vi "WrittingSpectrumAndImageAttributes.vi"() -> ()   [LabVIEW 2013, in "examples.lvlib"]
uses:
  examples.lvlib
  vis/lv-2013/tango_vi.llb/ReadULongImageAttribute.vi
  vis/lv-2013/tango_vi.llb/WriteULongImageAttribute.vi
  vis/lv-2013/tango_vi.llb/ReadDoubleImageAttribute.vi
  vis/lv-2013/tango_vi.llb/WriteDoubleImageAttribute.vi
  vis/lv-2013/tango_vi.llb/ReadFloatImageAttribute.vi
  vis/lv-2013/tango_vi.llb/WriteFloatImageAttribute.vi
  vis/lv-2013/tango_vi.llb/ReadBooleanImageAttribute.vi
  vis/lv-2013/tango_vi.llb/WriteBooleanImageAttribute.vi
  vis/lv-2013/tango_vi.llb/ReadUCharImageAttribute.vi
  vis/lv-2013/tango_vi.llb/WriteUCharImageAttribute.vi
  vis/lv-2013/tango_vi.llb/ReadUShortImageAttribute.vi
  vis/lv-2013/tango_vi.llb/WriteUShortImageAttribute.vi
  vis/lv-2013/tango_vi.llb/WriteLongSpectrumAttribute.vi
  vis/lv-2013/tango_vi.llb/ReadLongSpectrumAttribute.vi
  vis/lv-2013/tango_vi.llb/ReadLongImageAttribute.vi
  vis/lv-2013/tango_vi.llb/WriteLongImageAttribute.vi
  vis/lv-2013/tango_vi.llb/WriteDoubleSpectrumAttribute.vi
  vis/lv-2013/tango_vi.llb/ReadDoubleSpectrumAttribute.vi
  vis/lv-2013/tango_vi.llb/WriteFloatSpectrumAttribute.vi
  vis/lv-2013/tango_vi.llb/ReadFloatSpectrumAttribute.vi
  vis/lv-2013/tango_vi.llb/ReadShortImageAttribute.vi
  vis/lv-2013/tango_vi.llb/WriteShortImageAttribute.vi
  vis/lv-2013/tango_vi.llb/WriteUCharSpectrumAttribute.vi
  vis/lv-2013/tango_vi.llb/ReadUCharSpectrumAttribute.vi
  vis/lv-2013/tango_vi.llb/WriteBooleanSpectrumAttribute.vi
  vis/lv-2013/tango_vi.llb/ReadBooleanSpectrumAttribute.vi
  vis/lv-2013/tango_vi.llb/WriteUShortSpectrumAttribute.vi
  vis/lv-2013/tango_vi.llb/ReadUShortSpectrumAttribute.vi
  vis/lv-2013/tango_vi.llb/WriteShortSpectrumAttribute.vi
  vis/lv-2013/tango_vi.llb/ReadShortSpectrumAttribute.vi
  vis/lv-2013/tango_vi.llb/tango.lvlib
panel:
  in  "TangoTest dev. name 3":string="tango/tangotest/1"
  out "Success-R":bool
  out "Success-Cmp 3":bool
  out "ULong Image R":u32[][](graph)
  out "Success-W":bool
  out "ULong Image W":u32[][](graph)
  out "Success-R":bool
  out "Success-Cmp":bool
  out "Double  Image R":dbl[][](graph)
  out "Success-W":bool
  out "Double Image W":dbl[][](graph)
  out "Success-R":bool
  out "Success-Cmp":bool
  out "Float Image R":sgl[][](graph)
  out "Success-W":bool
  out "Float Image W":sgl[][](graph)
  out "Success-R":bool
  out "Success-Cmp":bool
  out "Boolean  Image R":i16[][](graph)
  out "Success-W":bool
  out "Boolean Image W":i16[][](graph)
  out "Success-R":bool
  out "Success-Cmp":bool
  out "UChar Image R":u8[][](graph)
  out "Success-W":bool
  out "UChar Image W":u8[][](graph)
  out "Success-R":bool
  out "Success-Cmp":bool
  out "UShort Image R":u16[][](graph)
  out "Success-W":bool
  out "UShort Image W":u16[][](graph)
  out "Long Spectrum R":i32[](graph)
  out "Success-R":bool
  out "Success-Cmp":bool
  out "Success-W":bool
  out "Long  Spectrum W":i32[](graph)
  out "Success-R":bool
  out "Success-Cmp":bool
  out "Long Image R":i32[][](graph)
  out "Success-W":bool
  out "Long Image W":i32[][](graph)
  out "Double Spectrum R":dbl[](graph)
  out "Success-R":bool
  out "Success-Cmp":bool
  out "Success-W":bool
  out "Double  Spectrum W":dbl[](graph)
  out "Float Spectrum R":sgl[](graph)
  out "Success-R":bool
  out "Success-Cmp":bool
  out "Success-W":bool
  out "Float Spectrum W":sgl[](graph)
  out "Short Image R":i16[][](graph)
  out "Short Image W":i16[][](graph)
  out "Success-R":bool
  out "Success-Cmp 2":bool
  out "Success-W":bool
  out "error stack":string[](array[string])
  in  "TangoTest Device Name 5":string="tango/tangotest/1"
  in  "TangoTest Device Name 4":string="tango/tangotest/1"
  in  "TangoTest Device Name 3":string="tango/tangotest/1"
  in  "TangoTest Device Name 2":string="tango/tangotest/1"
  in  "TangoTest dev. name":string="sys/tg_test/1"
  out "UChar Spectrum R":u8[](graph)
  out "Success-R":bool
  out "Success-Cmp":bool
  out "Success-W":bool
  out "UChar Spectrum W":u8[](graph)
  out "Boolean Spectrum R":i16[](graph)
  out "Success-R":bool
  out "Success-Cmp":bool
  out "Success-W":bool
  out "Boolean Spectrum W":i16[](graph)
  out "UShort Spectrum R":u16[](graph)
  out "Success-R":bool
  out "Success-Cmp":bool
  out "Success-W":bool
  out "UShort Spectrum W":u16[](graph)
  out "Success-Cmp":bool
  out "Success-W":bool
  out "Short Spectrum R":i16[](graph)
  out "Success-R":bool
  out "Short Spectrum W":i16[](graph)
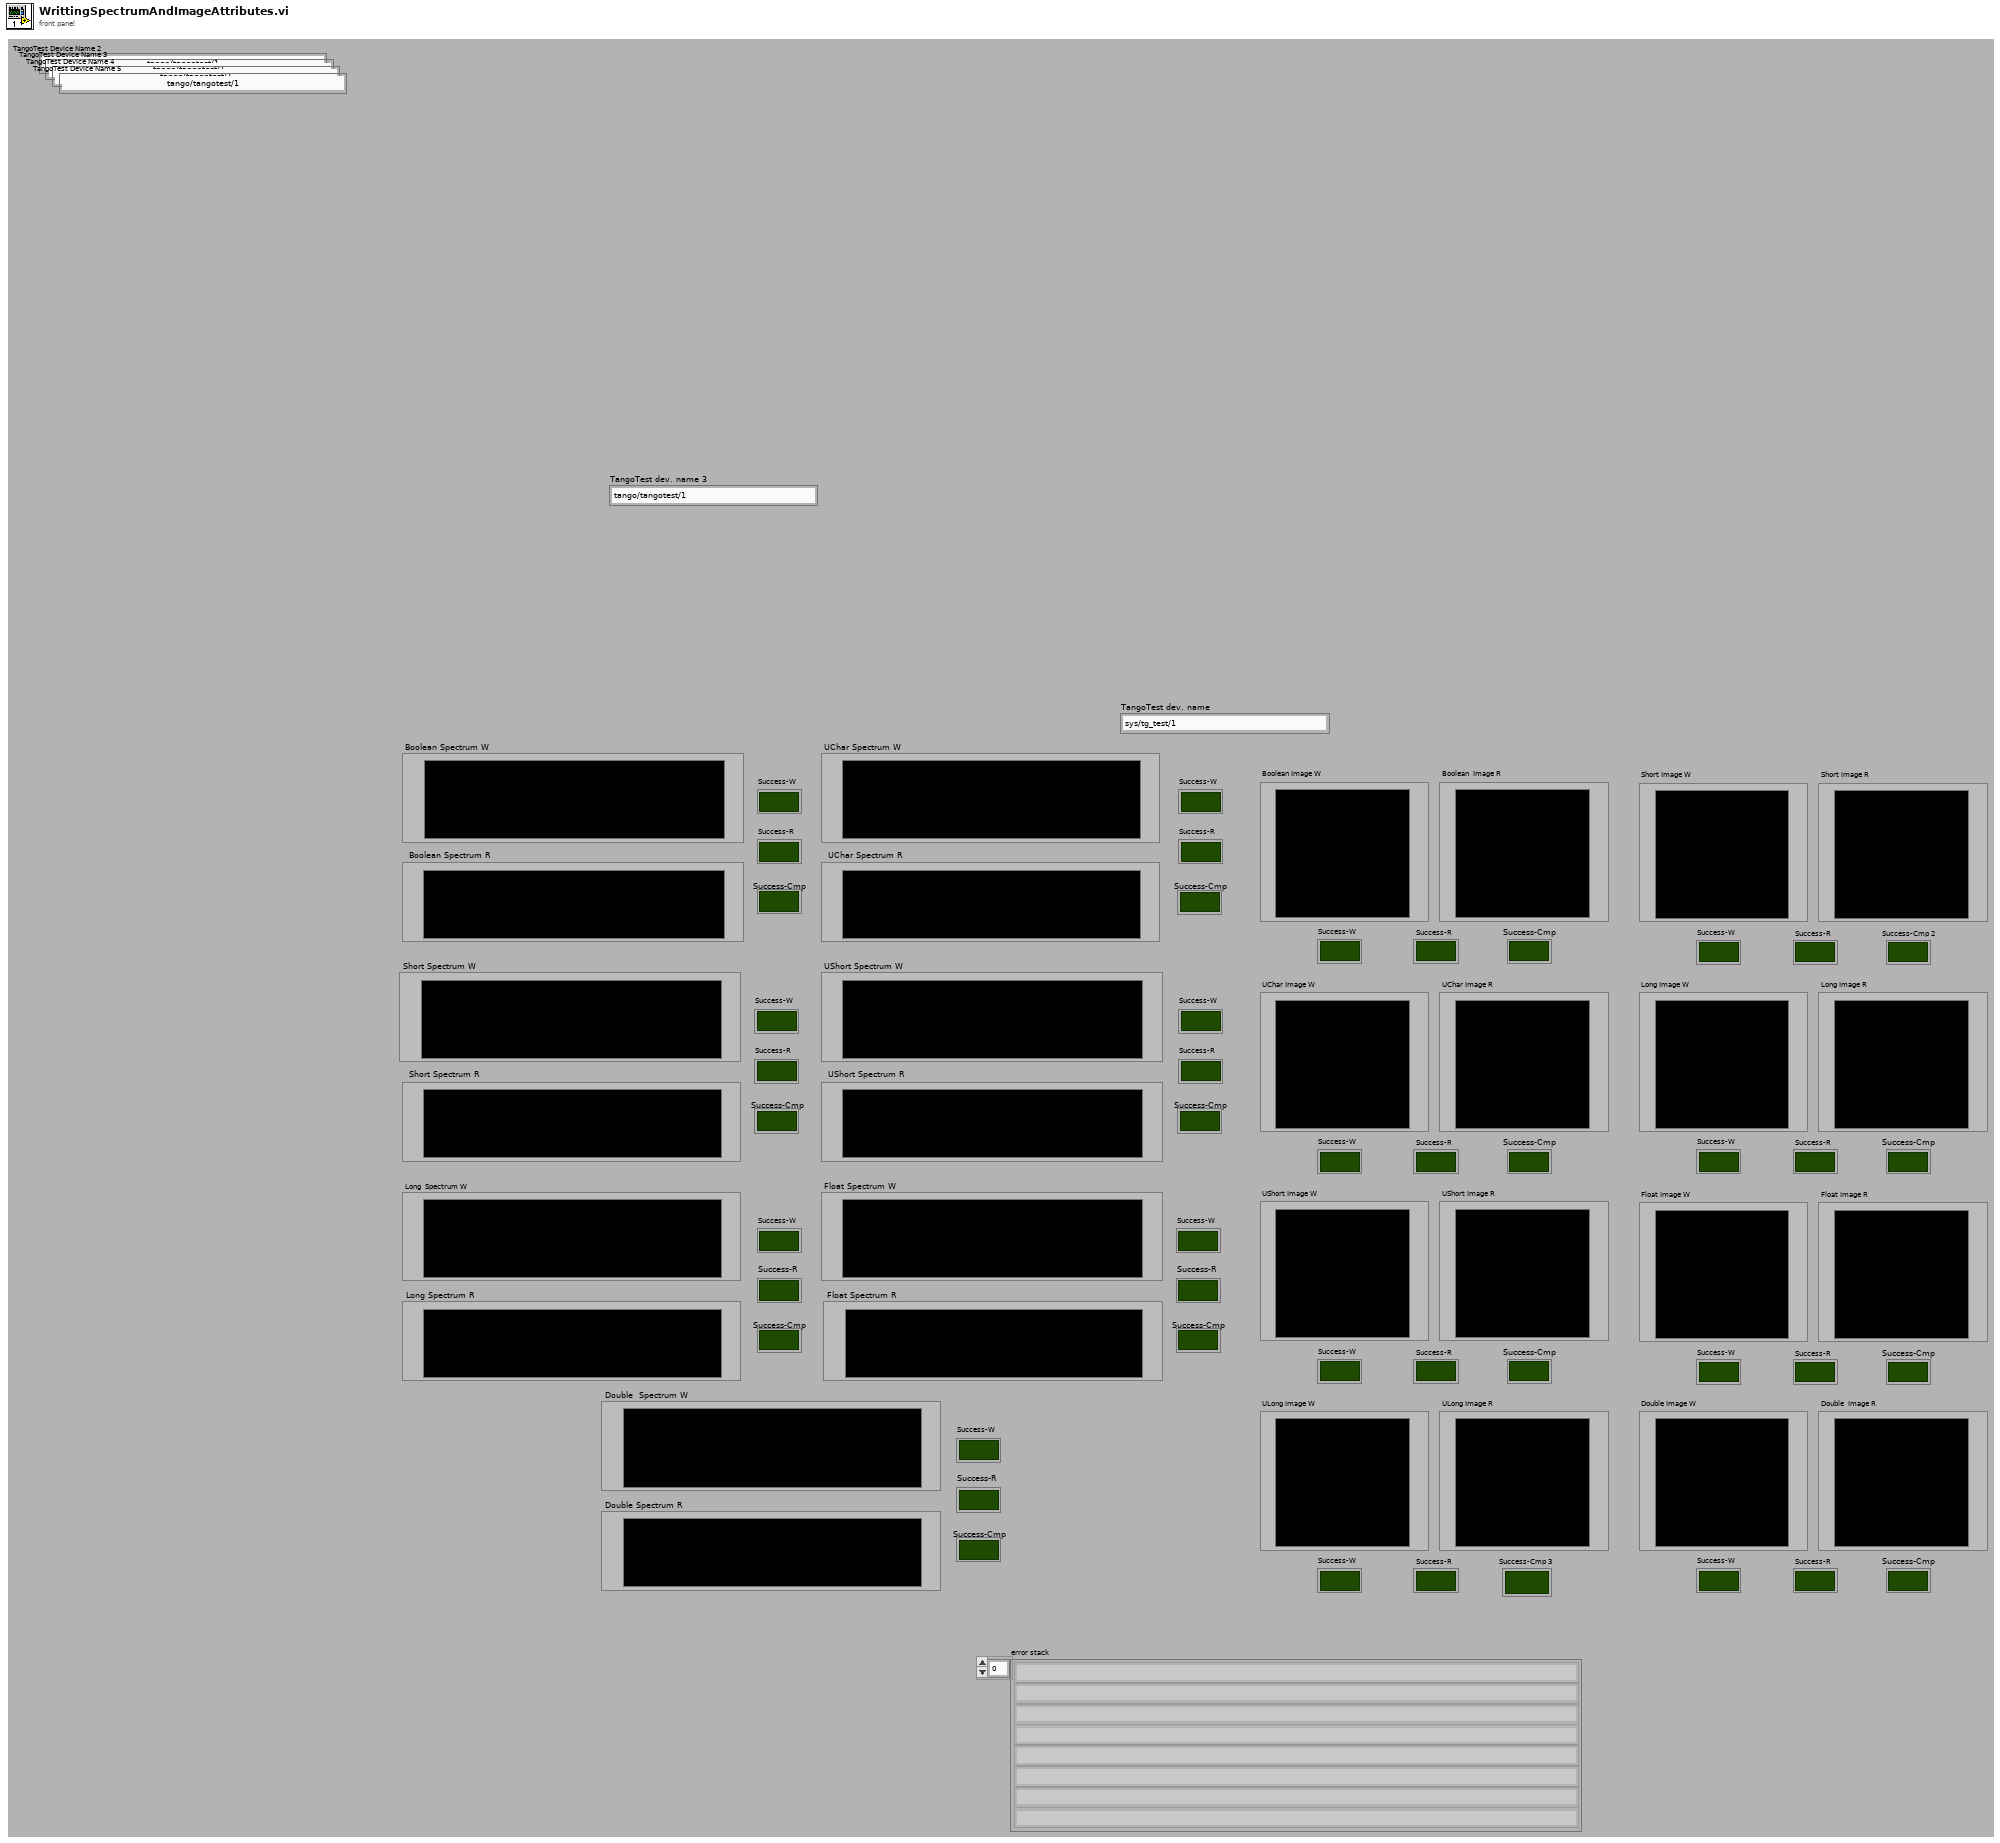
[diagram p1: front panel]
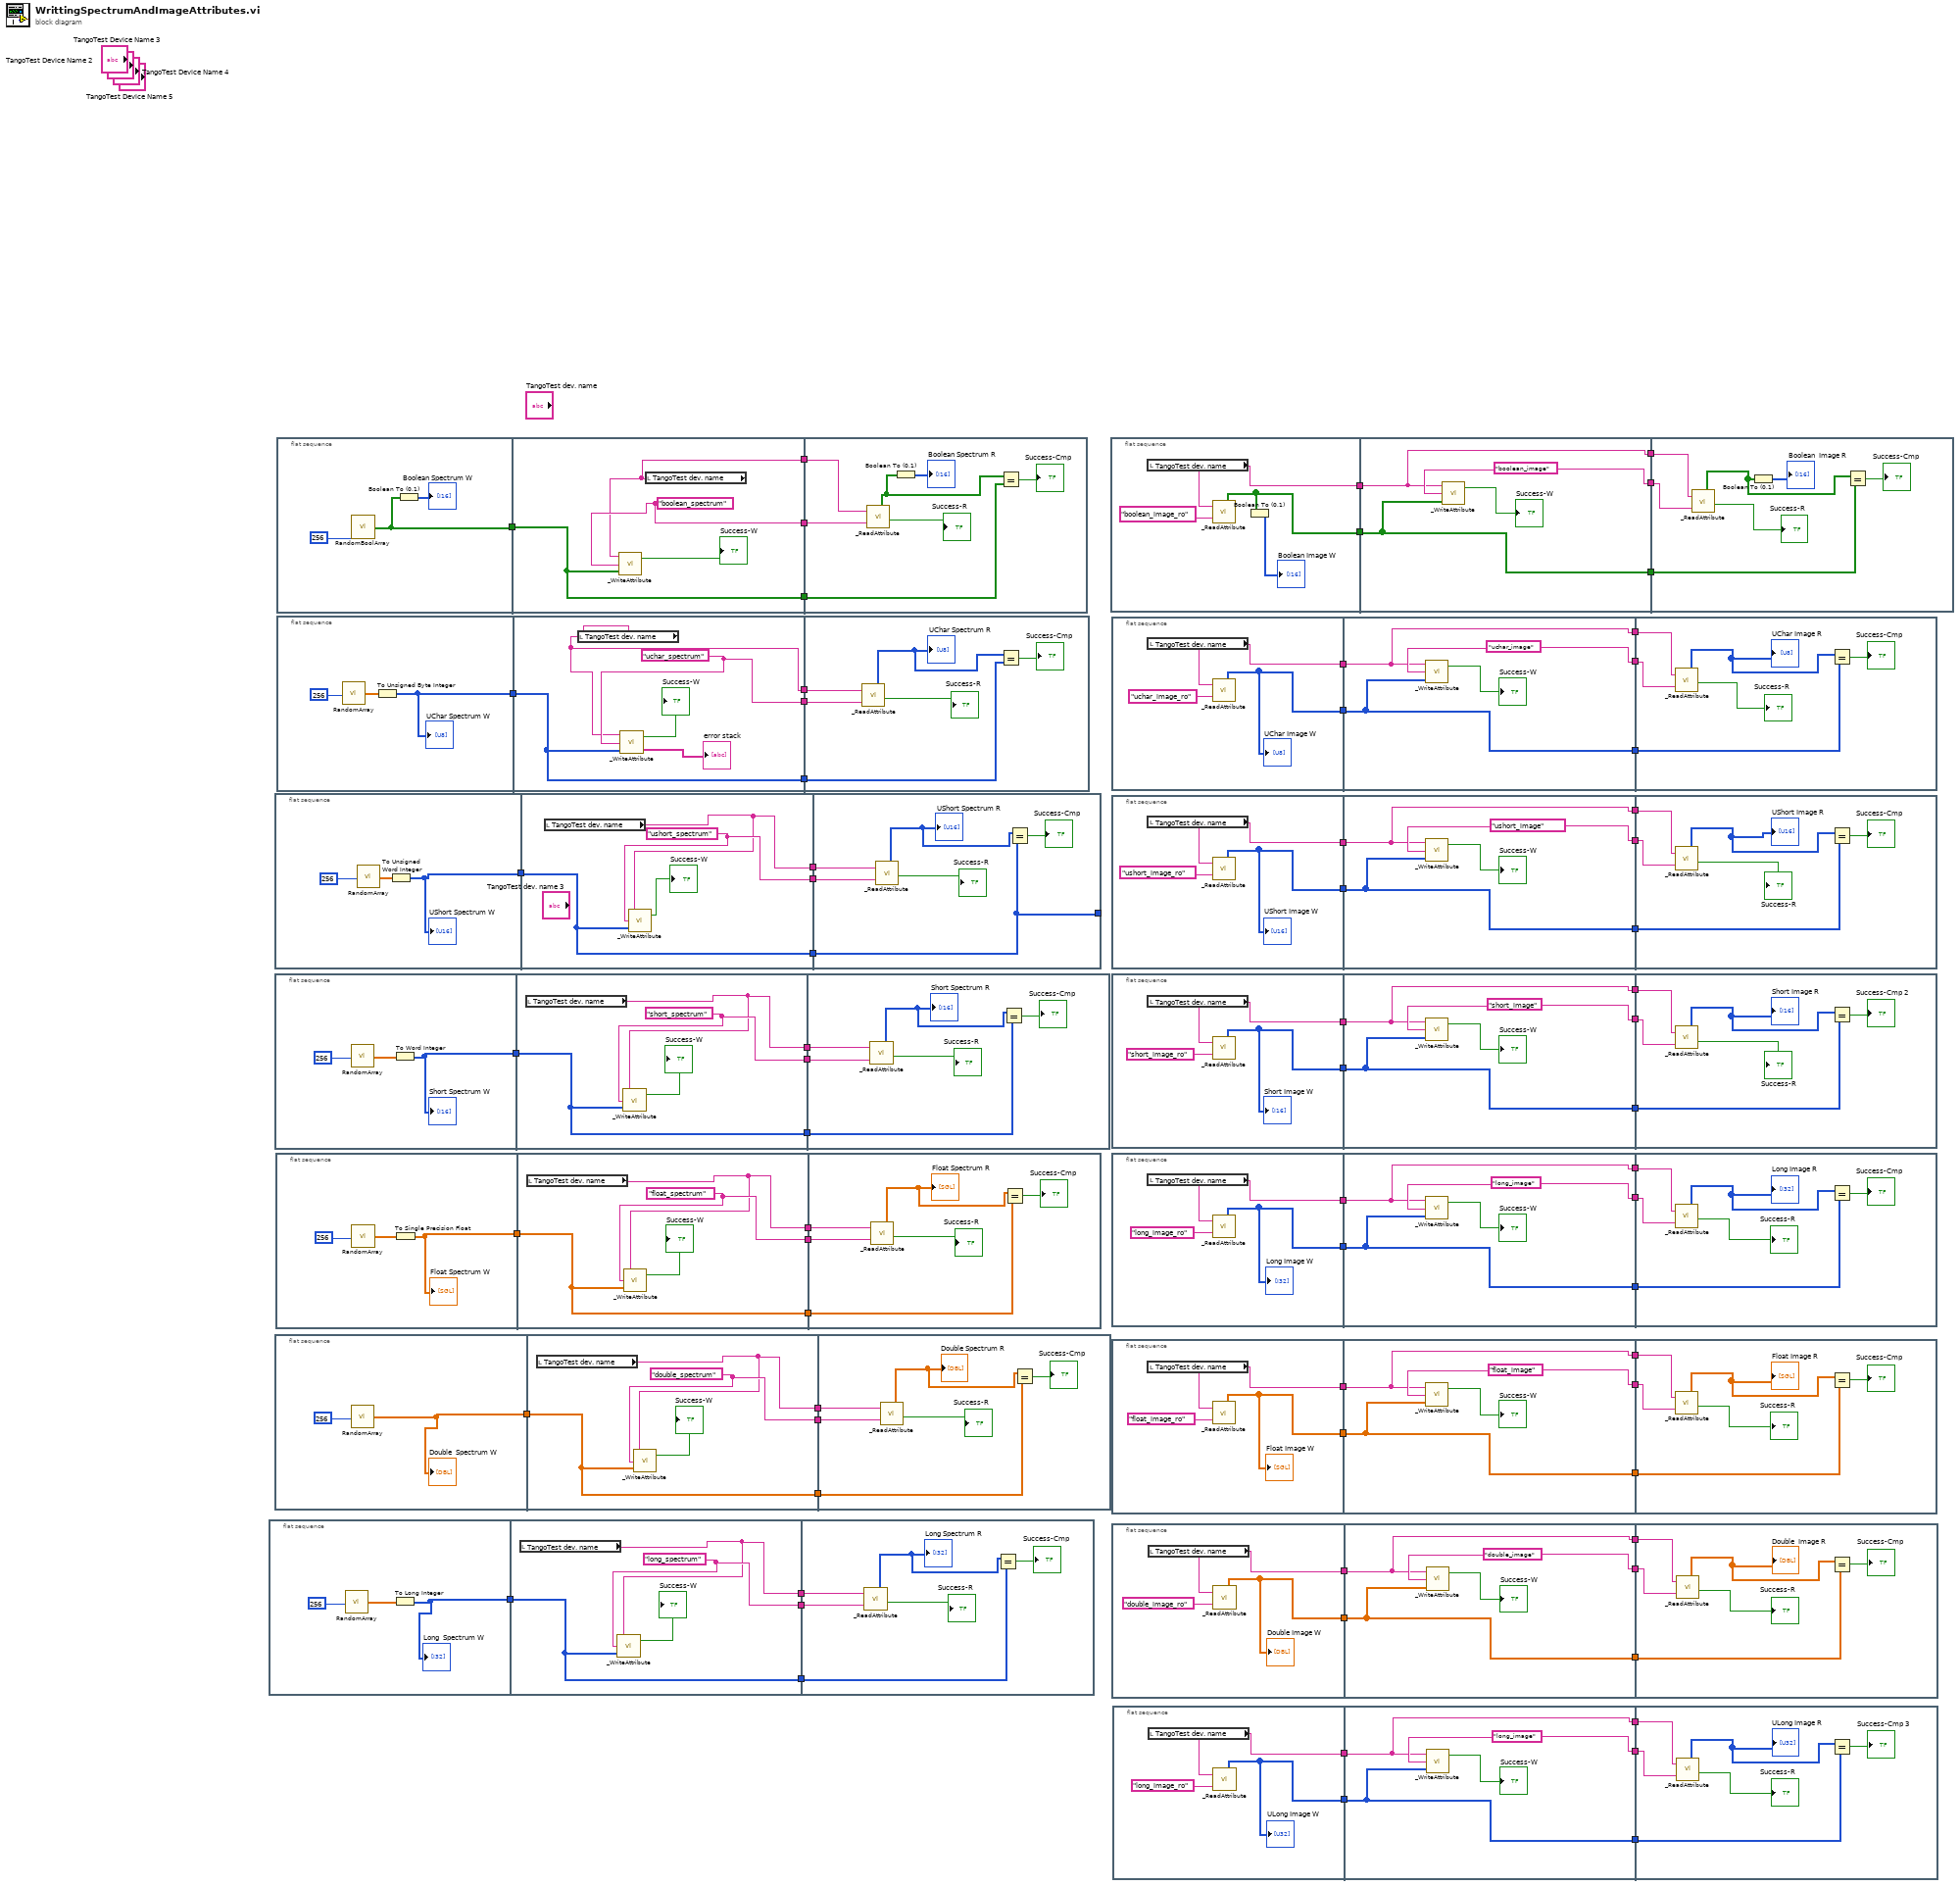
[diagram p0: block diagram]
diagram:
  n1 = flat-sequence {
    tunnel: [w69] -> w34
    tunnel: [w72] -> w33
    tunnel: [w74] -> w32
    tunnel: [w73] -> w31
    tunnel: w34 -> [w73]
    tunnel: w33 -> [w80]
    tunnel: w32 -> [w79]
    tunnel: w31 -> [w77]
    frame #0 {
      n2 = call "RandomArray.vi"("random array size"=256) -> ("random array"=w70:dbl[])  [unwired: 1 in]
      n3 = To Long Integer(number=w70) -> (32bit integer=w69:i32[])
      "Long  Spectrum W" <- w69
    }
    frame #1 {
      w74 = "long_spectrum" ("attribute name")
      n4 = local read "TangoTest dev. name"() -> (w72:string)
      n5 = call-poly "_WriteAttribute.vi"("value"=w73, "attribute name"=w74, "device name"=w72) -> ("success"=→"Success-W":bool)  [unwired: 1 out]
    }
    frame #2 {
      n6 = call-poly "_ReadAttribute.vi"("device name"=w80, "attribute name"=w79) -> ("value"=w78:i32[], "success"=→"Success-R":bool)  [unwired: 4 out]
      "Long Spectrum R" <- w78
      n7 = Equal?(x=w78, y=w77) -> (x = y?=→"Success-Cmp":bool)
    }
  }
  n8 = flat-sequence {
    tunnel: [w82] -> w64
    tunnel: [w86] -> w63
    tunnel: [w88] -> w62
    tunnel: [w87] -> w61
    tunnel: w64 -> [w87]
    tunnel: w63 -> [w93]
    tunnel: w62 -> [w92]
    tunnel: w61 -> [w89]
    tunnel: [w89] -> _
    frame #0 {
      n9 = call "RandomArray.vi"("random array size"=256) -> ("random array"=w83:dbl[])  [unwired: 1 in]
      n10 = To Unsigned Word Integer(number=w83) -> (unsigned 16bit integer=w82:u16[])
      "UShort Spectrum W" <- w82
    }
    frame #1 {
      w88 = "ushort_spectrum" ("attribute name")
      n11 = local read "TangoTest dev. name"() -> (w86:string)
      n12 = call-poly "_WriteAttribute.vi"("value"=w87, "attribute name"=w88, "device name"=w86) -> ("success"=→"Success-W":bool)  [unwired: 1 out]
    }
    frame #2 {
      n13 = call-poly "_ReadAttribute.vi"("device name"=w93, "attribute name"=w92) -> ("value"=w91:u16[], "success"=→"Success-R":bool)  [unwired: 4 out]
      "UShort Spectrum R" <- w91
      n14 = Equal?(x=w91, y=w89) -> (x = y?=→"Success-Cmp":bool)
    }
  }
  n15 = flat-sequence {
    tunnel: [w95] -> w65
    tunnel: [w98] -> w68
    tunnel: [w100] -> w67
    tunnel: [w99] -> w66
    tunnel: w65 -> [w99]
    tunnel: w68 -> [w106]
    tunnel: w67 -> [w105]
    tunnel: w66 -> [w103]
    frame #0 {
      n16 = call "RandomArray.vi"("random array size"=256) -> ("random array"=w96:dbl[])  [unwired: 1 in]
      n17 = To Word Integer(number=w96) -> (16bit integer=w95:i16[])
      "Short Spectrum W" <- w95
    }
    frame #1 {
      w100 = "short_spectrum" ("attribute name")
      n18 = local read "TangoTest dev. name"() -> (w98:string)
      n19 = call-poly "_WriteAttribute.vi"("value"=w99, "attribute name"=w100, "device name"=w98) -> ("success"=→"Success-W":bool)  [unwired: 1 out]
    }
    frame #2 {
      n20 = call-poly "_ReadAttribute.vi"("device name"=w106, "attribute name"=w105) -> ("value"=w104:i16[], "success"=→"Success-R":bool)  [unwired: 4 out]
      "Short Spectrum R" <- w104
      n21 = Equal?(x=w104, y=w103) -> (x = y?=→"Success-Cmp":bool)
    }
  }
  n22 = flat-sequence {
    tunnel: [w108] -> w43
    tunnel: [w110] -> w42
    tunnel: [w112] -> w41
    tunnel: [w111] -> w40
    tunnel: w43 -> [w111]
    tunnel: w42 -> [w118]
    tunnel: w41 -> [w117]
    tunnel: w40 -> [w115]
    frame #0 {
      n23 = call "RandomArray.vi"("random array size"=256) -> ("random array"=w108:dbl[])  [unwired: 1 in]
      "Double  Spectrum W" <- w108
    }
    frame #1 {
      w112 = "double_spectrum" ("attribute name")
      n24 = local read "TangoTest dev. name"() -> (w110:string)
      n25 = call-poly "_WriteAttribute.vi"("value"=w111, "attribute name"=w112, "device name"=w110) -> ("success"=→"Success-W":bool)  [unwired: 1 out]
    }
    frame #2 {
      n26 = call-poly "_ReadAttribute.vi"("device name"=w118, "attribute name"=w117) -> ("value"=w116:dbl[], "success"=→"Success-R":bool)  [unwired: 4 out]
      "Double Spectrum R" <- w116
      n27 = Equal?(x=w116, y=w115) -> (x = y?=→"Success-Cmp":bool)
    }
  }
  n28 = flat-sequence {
    tunnel: [w120] -> w47
    tunnel: [w123] -> w46
    tunnel: [w125] -> w45
    tunnel: [w124] -> w44
    tunnel: w47 -> [w124]
    tunnel: w46 -> [w131]
    tunnel: w45 -> [w130]
    tunnel: w44 -> [w128]
    frame #0 {
      n29 = call "RandomArray.vi"("random array size"=256) -> ("random array"=w121:dbl[])  [unwired: 1 in]
      n30 = To Single Precision Float(number=w121) -> (single precision float=w120:sgl[])
      "Float Spectrum W" <- w120
    }
    frame #1 {
      w125 = "float_spectrum" ("attribute name")
      n31 = local read "TangoTest dev. name"() -> (w123:string)
      n32 = call-poly "_WriteAttribute.vi"("value"=w124, "attribute name"=w125, "device name"=w123) -> ("success"=→"Success-W":bool)  [unwired: 1 out]
    }
    frame #2 {
      n33 = call-poly "_ReadAttribute.vi"("device name"=w131, "attribute name"=w130) -> ("value"=w129:sgl[], "success"=→"Success-R":bool)  [unwired: 4 out]
      "Float Spectrum R" <- w129
      n34 = Equal?(x=w129, y=w128) -> (x = y?=→"Success-Cmp":bool)
    }
  }
  n35 = flat-sequence {
    tunnel: [w133] -> w54
    tunnel: [w137] -> w58
    tunnel: [w139] -> w57
    tunnel: w54 -> [w138]
    tunnel: [w138] -> w53
    tunnel: w58 -> [w145]
    tunnel: w57 -> [w144]
    tunnel: w53 -> [w141]
    frame #0 {
      n36 = call "RandomArray.vi"("random array size"=256) -> ("random array"=w134:dbl[])  [unwired: 1 in]
      n37 = To Unsigned Byte Integer(number=w134) -> (unsigned 8bit integer=w133:u8[])
      "UChar Spectrum W" <- w133
    }
    frame #1 {
      w139 = "uchar_spectrum" ("attribute name")
      n38 = local read "TangoTest dev. name"() -> (w137:string)
      n39 = call-poly "_WriteAttribute.vi"("value"=w138, "attribute name"=w139, "device name"=w137) -> ("error stack"=→"error stack":string[], "success"=→"Success-W":bool)
    }
    frame #2 {
      n40 = call-poly "_ReadAttribute.vi"("device name"=w145, "attribute name"=w144) -> ("value"=w143:u8[], "success"=→"Success-R":bool)  [unwired: 4 out]
      "UChar Spectrum R" <- w143
      n41 = Equal?(x=w143, y=w141) -> (x = y?=→"Success-Cmp":bool)
    }
  }
  n42 = flat-sequence {
    tunnel: [w148] -> w60
    tunnel: [w152] -> w59
    tunnel: w60 -> [w152]
    tunnel: [w151] -> w56
    tunnel: [w150] -> w55
    tunnel: w59 -> [w156]
    tunnel: w56 -> [w155]
    tunnel: w55 -> [w154]
    frame #0 {
      n43 = call "RandomBoolArray.vi"("random array size"=256) -> ("random array"=w148:bool[])  [unwired: 1 in]
      n44 = Boolean To (0,1)(Boolean=w148) -> (0, 1=→"Boolean Spectrum W":i16[])
    }
    frame #1 {
      w151 = "boolean_spectrum" ("attribute name")
      n45 = local read "TangoTest dev. name"() -> (w150:string)
      n46 = call-poly "_WriteAttribute.vi"("value"=w152, "attribute name"=w151, "device name"=w150) -> ("success"=→"Success-W":bool)  [unwired: 1 out]
    }
    frame #2 {
      n47 = call-poly "_ReadAttribute.vi"("device name"=w154, "attribute name"=w155) -> ("value"=w158:bool[], "success"=→"Success-R":bool)  [unwired: 4 out]
      n48 = Boolean To (0,1)(Boolean=w158) -> (0, 1=→"Boolean Spectrum R":i16[])
      n49 = Equal?(x=w158, y=w156) -> (x = y?=→"Success-Cmp":bool)
    }
  }
  n50 = flat-sequence {
    tunnel: [w163] -> w20
    tunnel: [w162] -> w19
    tunnel: [w168] -> w18
    tunnel: [w166] -> w17
    tunnel: w20 -> [w166]
    tunnel: w19 -> [w165]
    tunnel: [w165] -> w16
    tunnel: w18 -> [w174]
    tunnel: w17 -> [w171]
    tunnel: w16 -> [w170]
    frame #0 {
      n51 = local read "TangoTest dev. name"() -> (w162:string)
      n52 = call-poly "_ReadAttribute.vi"("device name"=w162, "attribute name"="boolean_image_ro") -> ("value"=w163:bool[][])  [unwired: 5 out]
      n53 = Boolean To (0,1)(Boolean=w163) -> (0, 1=→"Boolean Image W":i16[][])
    }
    frame #1 {
      w168 = "boolean_image" ("attribute name")
      n54 = call-poly "_WriteAttribute.vi"("value"=w166, "attribute name"=w168, "device name"=w165) -> ("success"=→"Success-W":bool)  [unwired: 1 out]
    }
    frame #2 {
      n55 = call-poly "_ReadAttribute.vi"("device name"=w170, "attribute name"=w174) -> ("value"=w172:bool[][], "success"=→"Success-R":bool)  [unwired: 4 out]
      n56 = Boolean To (0,1)(Boolean=w172) -> (0, 1=→"Boolean  Image R":i16[][])
      n57 = Equal?(x=w172, y=w171) -> (x = y?=→"Success-Cmp":bool)
    }
  }
  n58 = flat-sequence {
    tunnel: [w177] -> w25
    tunnel: [w176] -> w24
    tunnel: [w182] -> w23
    tunnel: [w180] -> w22
    tunnel: w25 -> [w180]
    tunnel: w24 -> [w179]
    tunnel: [w179] -> w21
    tunnel: w23 -> [w187]
    tunnel: w22 -> [w184]
    tunnel: w21 -> [w183]
    frame #0 {
      n59 = local read "TangoTest dev. name"() -> (w176:string)
      n60 = call-poly "_ReadAttribute.vi"("device name"=w176, "attribute name"="uchar_image_ro") -> ("value"=w177:u8[][])  [unwired: 5 out]
      "UChar Image W" <- w177
    }
    frame #1 {
      w182 = "uchar_image" ("attribute name")
      n61 = call-poly "_WriteAttribute.vi"("value"=w180, "attribute name"=w182, "device name"=w179) -> ("success"=→"Success-W":bool)  [unwired: 1 out]
    }
    frame #2 {
      n62 = call-poly "_ReadAttribute.vi"("device name"=w183, "attribute name"=w187) -> ("value"=w185:u8[][], "success"=→"Success-R":bool)  [unwired: 4 out]
      "UChar Image R" <- w185
      n63 = Equal?(x=w185, y=w184) -> (x = y?=→"Success-Cmp":bool)
    }
  }
  n64 = flat-sequence {
    tunnel: [w190] -> w30
    tunnel: [w189] -> w29
    tunnel: [w195] -> w28
    tunnel: [w193] -> w27
    tunnel: w30 -> [w193]
    tunnel: w29 -> [w192]
    tunnel: [w192] -> w26
    tunnel: w28 -> [w200]
    tunnel: w27 -> [w198]
    tunnel: w26 -> [w197]
    frame #0 {
      n65 = local read "TangoTest dev. name"() -> (w189:string)
      n66 = call-poly "_ReadAttribute.vi"("device name"=w189, "attribute name"="ushort_image_ro") -> ("value"=w190:u16[][])  [unwired: 5 out]
      "UShort Image W" <- w190
    }
    frame #1 {
      w195 = "ushort_image" ("attribute name")
      n67 = call-poly "_WriteAttribute.vi"("value"=w193, "attribute name"=w195, "device name"=w192) -> ("success"=→"Success-W":bool)  [unwired: 1 out]
    }
    frame #2 {
      n68 = call-poly "_ReadAttribute.vi"("device name"=w197, "attribute name"=w200) -> ("value"=w196:u16[][], "success"=→"Success-R":bool)  [unwired: 4 out]
      "UShort Image R" <- w196
      n69 = Equal?(x=w196, y=w198) -> (x = y?=→"Success-Cmp":bool)
    }
  }
  n70 = flat-sequence {
    tunnel: [w203] -> w50
    tunnel: [w202] -> w49
    tunnel: [w208] -> w52
    tunnel: [w206] -> w51
    tunnel: w50 -> [w206]
    tunnel: w49 -> [w205]
    tunnel: [w205] -> w48
    tunnel: w52 -> [w213]
    tunnel: w51 -> [w210]
    tunnel: w48 -> [w209]
    frame #0 {
      n71 = local read "TangoTest dev. name"() -> (w202:string)
      n72 = call-poly "_ReadAttribute.vi"("device name"=w202, "attribute name"="short_image_ro") -> ("value"=w203:i16[][])  [unwired: 5 out]
      "Short Image W" <- w203
    }
    frame #1 {
      w208 = "short_image" ("attribute name")
      n73 = call-poly "_WriteAttribute.vi"("value"=w206, "attribute name"=w208, "device name"=w205) -> ("success"=→"Success-W":bool)  [unwired: 1 out]
    }
    frame #2 {
      n74 = call-poly "_ReadAttribute.vi"("device name"=w209, "attribute name"=w213) -> ("value"=w211:i16[][], "success"=→"Success-R":bool)  [unwired: 4 out]
      "Short Image R" <- w211
      n75 = Equal?(x=w211, y=w210) -> (x = y?=→"Success-Cmp 2":bool)
    }
  }
  n76 = flat-sequence {
    tunnel: [w216] -> w39
    tunnel: [w215] -> w38
    tunnel: [w221] -> w37
    tunnel: [w219] -> w36
    tunnel: w39 -> [w219]
    tunnel: w38 -> [w218]
    tunnel: [w218] -> w35
    tunnel: w37 -> [w226]
    tunnel: w36 -> [w223]
    tunnel: w35 -> [w222]
    frame #0 {
      n77 = local read "TangoTest dev. name"() -> (w215:string)
      n78 = call-poly "_ReadAttribute.vi"("device name"=w215, "attribute name"="long_image_ro") -> ("value"=w216:i32[][])  [unwired: 5 out]
      "Long Image W" <- w216
    }
    frame #1 {
      w221 = "long_image" ("attribute name")
      n79 = call-poly "_WriteAttribute.vi"("value"=w219, "attribute name"=w221, "device name"=w218) -> ("success"=→"Success-W":bool)  [unwired: 1 out]
    }
    frame #2 {
      n80 = call-poly "_ReadAttribute.vi"("device name"=w222, "attribute name"=w226) -> ("value"=w224:i32[][], "success"=→"Success-R":bool)  [unwired: 4 out]
      "Long Image R" <- w224
      n81 = Equal?(x=w224, y=w223) -> (x = y?=→"Success-Cmp":bool)
    }
  }
  n82 = flat-sequence {
    tunnel: [w229] -> w15
    tunnel: [w228] -> w14
    tunnel: [w234] -> w13
    tunnel: [w232] -> w12
    tunnel: w15 -> [w232]
    tunnel: w14 -> [w231]
    tunnel: [w231] -> w11
    tunnel: w13 -> [w239]
    tunnel: w12 -> [w236]
    tunnel: w11 -> [w235]
    frame #0 {
      n83 = local read "TangoTest dev. name"() -> (w228:string)
      n84 = call-poly "_ReadAttribute.vi"("device name"=w228, "attribute name"="float_image_ro") -> ("value"=w229:sgl[][])  [unwired: 5 out]
      "Float Image W" <- w229
    }
    frame #1 {
      w234 = "float_image" ("attribute name")
      n85 = call-poly "_WriteAttribute.vi"("value"=w232, "attribute name"=w234, "device name"=w231) -> ("success"=→"Success-W":bool)  [unwired: 1 out]
    }
    frame #2 {
      n86 = call-poly "_ReadAttribute.vi"("device name"=w235, "attribute name"=w239) -> ("value"=w237:sgl[][], "success"=→"Success-R":bool)  [unwired: 4 out]
      "Float Image R" <- w237
      n87 = Equal?(x=w237, y=w236) -> (x = y?=→"Success-Cmp":bool)
    }
  }
  n88 = flat-sequence {
    tunnel: [w242] -> w10
    tunnel: [w241] -> w9
    tunnel: [w247] -> w8
    tunnel: [w245] -> w7
    tunnel: w10 -> [w245]
    tunnel: w9 -> [w244]
    tunnel: [w244] -> w6
    tunnel: w8 -> [w252]
    tunnel: w7 -> [w249]
    tunnel: w6 -> [w248]
    frame #0 {
      n89 = local read "TangoTest dev. name"() -> (w241:string)
      n90 = call-poly "_ReadAttribute.vi"("device name"=w241, "attribute name"="double_image_ro") -> ("value"=w242:dbl[][])  [unwired: 5 out]
      "Double Image W" <- w242
    }
    frame #1 {
      w247 = "double_image" ("attribute name")
      n91 = call-poly "_WriteAttribute.vi"("value"=w245, "attribute name"=w247, "device name"=w244) -> ("success"=→"Success-W":bool)  [unwired: 1 out]
    }
    frame #2 {
      n92 = call-poly "_ReadAttribute.vi"("device name"=w248, "attribute name"=w252) -> ("value"=w250:dbl[][], "success"=→"Success-R":bool)  [unwired: 4 out]
      "Double  Image R" <- w250
      n93 = Equal?(x=w250, y=w249) -> (x = y?=→"Success-Cmp":bool)
    }
  }
  n94 = flat-sequence {
    tunnel: [w255] -> w5
    tunnel: [w254] -> w4
    tunnel: [w260] -> w3
    tunnel: [w258] -> w2
    tunnel: w5 -> [w258]
    tunnel: w4 -> [w257]
    tunnel: [w257] -> w1
    tunnel: w3 -> [w265]
    tunnel: w2 -> [w262]
    tunnel: w1 -> [w261]
    frame #0 {
      n95 = local read "TangoTest dev. name"() -> (w254:string)
      n96 = call-poly "_ReadAttribute.vi"("device name"=w254, "attribute name"="long_image_ro") -> ("value"=w255:u32[][])  [unwired: 5 out]
      "ULong Image W" <- w255
    }
    frame #1 {
      w260 = "long_image" ("attribute name")
      n97 = call-poly "_WriteAttribute.vi"("value"=w258, "attribute name"=w260, "device name"=w257) -> ("success"=→"Success-W":bool)  [unwired: 1 out]
    }
    frame #2 {
      n98 = call-poly "_ReadAttribute.vi"("device name"=w261, "attribute name"=w265) -> ("value"=w263:u32[][], "success"=→"Success-R":bool)  [unwired: 4 out]
      "ULong Image R" <- w263
      n99 = Equal?(x=w263, y=w262) -> (x = y?=→"Success-Cmp 3":bool)
    }
  }
